vi "CSDB_Config.set Database.vi"(5 "error in (no error)":errorcluster) -> (15 "Database":string, 19 "error out":errorcluster)   [LabVIEW 2014, in "CSDB_Config.lvlib"]
doc: "Sets the database which is to be configured"
uses:
  CSDB_Config.lvlib
  <vilib>/addons/database/Connection.llb/DB Tools Open Connec (String).vi
  <vilib>/addons/database/NI_Database_API.lvlib
panel:
  in  "OK Button":bool
  in  "Database (default = Process)":string="Process"
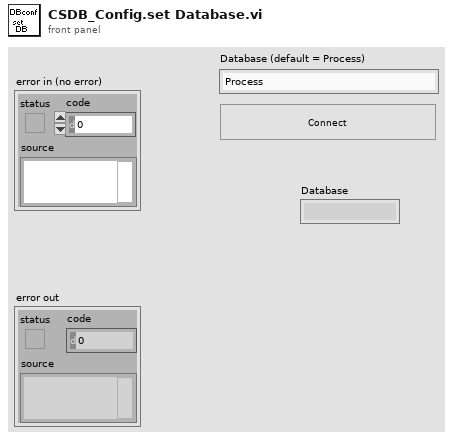
[diagram p1: front panel]
types:
  T1 = typedef "NI_Database_API.lvlib/Conn ObjectReference.ctl" = refnum<k1>
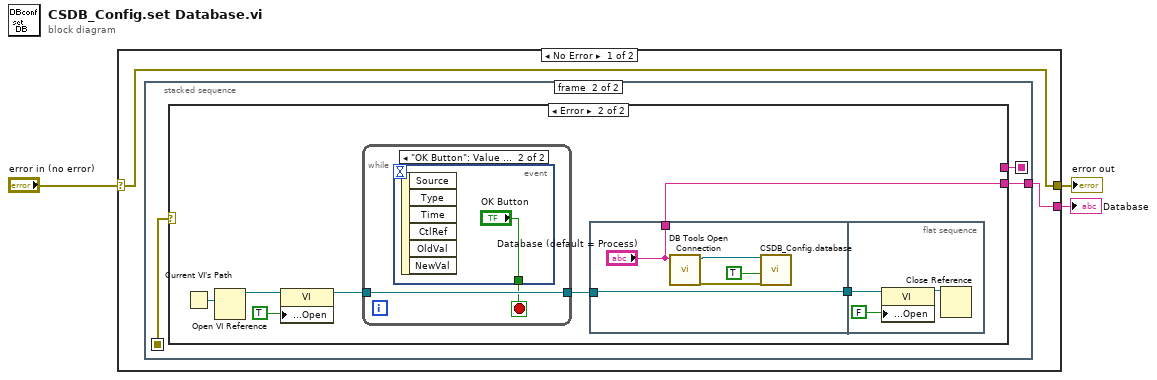
[diagram p0: block diagram]
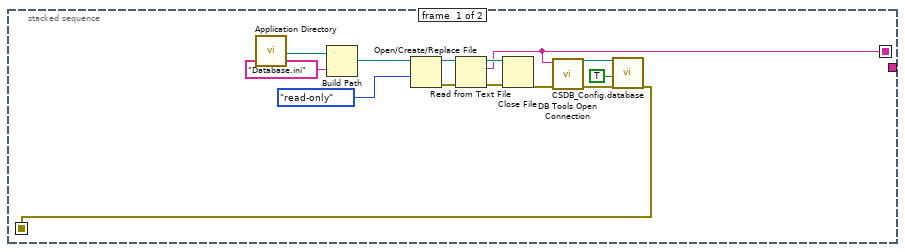
[diagram p2: hidden frame]
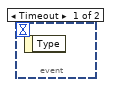
[diagram p4: hidden frame]
diagram:
  n1 = case shown="No Error" "error in (no error)" {
    selector: "error in (no error)" -> [w5 w42]
    tunnel: [w5 w42] -> w3
    tunnel: [w4 _] -> w1
    frame No Error {
      n2 = stacked-sequence {
        seq-local: [w7 _] -> [_ w22]
        seq-local: [w6 _] -> [_ w21]
        tunnel: [_ w20] -> w4
        frame #0 {
          n3 = call <vilib>:"Application Directory.vi"() -> ("Application Directory"=w19:path)
          n4 = Build Path(base path=w19, name or relative path="Database.ini") -> (appended path=w17:path)
          n5 = Open/Create/Replace File(file path (use dialog)=w17, access (0:read/write)=enum16{"read/write", "read-only", "write-only"}."read-only") -> (refnum out=w11:refnum<file>, error out=w12:errorcluster)  [unwired: 4 in, 1 out]
          n6 = Read from Text File(file (use dialog)=w11, error in=w12) -> (refnum out=w9:refnum<file>, text=w6:string, error out=w10:errorcluster)  [unwired: 2 in, 1 out]
          n7 = Close File(refnum=w9, error in=w10) -> (error out=w8:errorcluster)  [unwired: 1 out]
          n8 = call-poly <vilib>:"DB Tools Open Connection.vi"("error in (no error)"=w8, "connection information"=w6) -> ("error out"=w14:errorcluster, "connection reference"=w15:T1)  [unwired: 6 in]
          n9 = call "CSDB_Config.database.vi"("connectionRef"=w15, "setReference"=TRUE, "error in (no error)"=w14) -> ("error out"=w7:errorcluster)  [unwired: 15 in, 1 out]
        }
        frame #1 {
          n10 = case shown="Error" w22 {
            tunnel: [w23 w24] -> w20
            tunnel: w21 -> [w23 _]
            frame No Error {
            }
            frame Error {
              n11 = Current VI's Path() -> (path=w29:path)
              n12 = Open VI Reference(vi path=w29) -> (vi reference=w28:refnum<vi>)  [unwired: 5 in, 1 out]
              n13 = property class="VI"(reference=w28, "Front Panel Window:Open"=TRUE) -> (reference out=w26:refnum<vi>)  [unwired: 1 in, 1 out]
              n14 = while {
                tunnel: [w40] -> w25
                tunnel: w26 -> [w40]
                stop <- w39 stop-if-true
                n15 = event shown="[1] \"OK Button\": Value Change" {
                  selector: _ -> [_ _]
                  dyn-events: _ -> [_ _]
                  timeout: _ -> [_ _]
                  tunnel: [_ "OK Button"] -> w39
                  event Timeout {
                    n16 = event-data() -> ()  [unwired: 1 in, 1 out]
                  }
                  event "OK Button": Value Change {
                    n17 = event-data() -> ()  [unwired: 1 in, 6 out]
                  }
                }
              }
              n18 = flat-sequence {
                tunnel: w25 -> [w35]
                tunnel: [w35] -> w30
                tunnel: ["Database (default = Process)"] -> w24
                tunnel: w30 -> [w38]
                frame #0 {
                  n19 = call-poly <vilib>:"DB Tools Open Connection.vi"("connection information"="Database (default = Process)") -> ("error out"=w33:errorcluster, "connection reference"=w34:T1)  [unwired: 7 in]
                  n20 = call "CSDB_Config.database.vi"("connectionRef"=w34, "setReference"=TRUE, "error in (no error)"=w33) -> ()  [unwired: 15 in, 2 out]
                }
                frame #1 {
                  n21 = property class="VI"(reference=w38, "Front Panel Window:Open"=FALSE) -> (reference out=w36:refnum<vi>)  [unwired: 1 in, 1 out]
                  n22 = Close Reference(reference=w36) -> ()  [unwired: 1 in, 1 out]
                }
              }
            }
          }
        }
      }
    }
    frame Error {
    }
  }
  "error out" <- w3
  "Database" <- w1
